vi "send load report.vi"(8 "error in":errorcluster, 9 "load error":errorcluster, 10 "engine loaded":string, 11 "message queue in":T1) -> (0 "error out":errorcluster, 3 "message queue out":T1)   [LabVIEW 2013, in "module execution process.lvlib"]
uses:
  module execution process.lvlib
  <vilib>/NI/AMC/Message Queue.ctl
  <vilib>/NI/AMC/Message.ctl
  <vilib>/NI/Tools/Keyed Array/KeyedArray.ctl
  common reponses to network process.ctl
  <vilib>/NI/AMC/Create Single Message.vi
  <vilib>/NI/AMC/Update Message Routing Info.vi
  <vilib>/NI/AMC/Send Message.vi
  <vilib>/NI/AMC/AMC.lvlib
  <vilib>/NI/Tools/Keyed Array/Tools_KeyedArray.lvlib
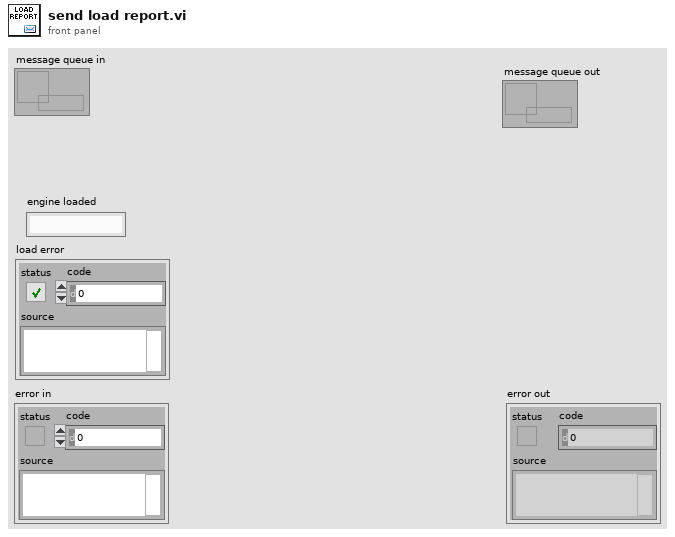
[diagram p1: front panel]
types:
  T1 = typedef "AMC.lvlib/Message Queue.ctl" = refnum<queue>
  T2 = typedef "module execution process.lvlib/common reponses to network process.ctl" = enum16{"System Error", "Load Report", "Action Response", "Engine Status"}
  T3 = cluster{"engine loaded":string, "load error":errorcluster}
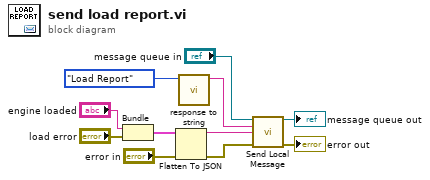
[diagram p0: block diagram]
diagram:
  n1 = Bundle("engine loaded"="engine loaded", "load error"="load error") -> (w5:T3)  [unwired: 1 in]
  n2 = Flatten To JSON(anything=w5, error in (no error)="error in") -> (JSON string=w6:string, 11:w7:errorcluster)  [unwired: 1 in]
  n3 = call "response to string.vi"("responses"=common_reponses_to_network_process."Load Report") -> ("command string"=w2:string)  [unwired: 10 in]
  n4 = call <vilib>:"Send Local Message.vi"("message queue in"="message queue in", "message name"=w2, "message value"=w6, "error in"=w7) -> ("message queue out"=→"message queue out":T1, "error out"=→"error out":errorcluster)  [unwired: 9 in, 1 out]
